vi "Read String.vi"(7 "count (-1: rest)":i64=-1 format="%d elements", 8 "error in (no error)":errorcluster, 9 "offset (0)":u64 format="%d bytes", 10 "buffer in":string, 11 "Pointer in":refnum<class "Pointer.lvclass">) -> (0 "error out":errorcluster, 1 "offset out":u64 format="%d bytes", 2 "buffer out":string, 3 "Pointer out":refnum<class "Pointer.lvclass">)   [LabVIEW 2027, in "Memory Manager.lvlib" / "Pointer.lvclass"]
doc: "Reads <b>count</b> bytes from the address specified by <b>pointer + offset</b> into the provided <b>buffer</b>."
uses:
  Pointer.lvclass
  Read (No Check) String.vi
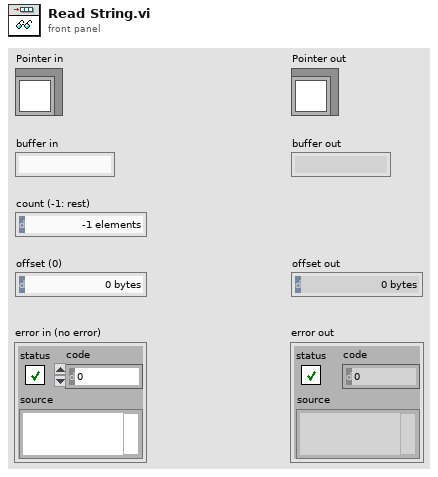
[diagram p1: front panel]
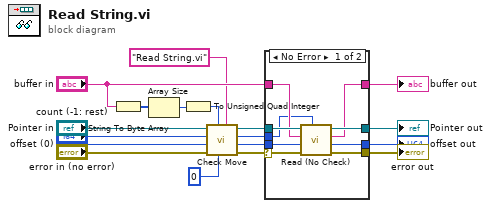
[diagram p0: block diagram]
diagram:
  n1 = String To Byte Array(string="buffer in") -> (unsigned byte array=w14:u8[])
  n2 = Array Size(array=w14) -> (size(s)=w13:i32)
  n3 = To Unsigned Quad Integer(1:w13) -> (0:w7:u64)
  n4 = call "Check Move.vi"("source vi name"="Read String.vi", "count power of 2"=u8 0, "buffer count"=w7, "error in (no error)"="error in (no error)", "offset (0)"="offset (0)", "move count (-1: rest)"="count (-1: rest)", "Pointer in"="Pointer in") -> ("error out"=w10:errorcluster, "offset"=w9:u64, "count"=w8:u64, "Pointer out"=w11:refnum<class "Pointer.lvclass">)  [unwired: 1 in]
  n5 = case shown="No Error" w10 {
    selector: w10 -> [w27 w30]
    tunnel: w11 -> [w25 w29]
    tunnel: w9 -> [w26 w31]
    tunnel: "buffer in" -> [w20 w28]
    tunnel: [w24 w30] -> w18
    tunnel: [w23 w29] -> w16
    tunnel: [w22 w31] -> w15
    tunnel: [w21 w28] -> w17
    tunnel: w8 -> [w19 _]
    frame No Error {
      n6 = call-poly "Read (No Check).vi"("count"=w19, "error in (no error)"=w27, "offset (0)"=w26, "buffer in"=w20, "Pointer in"=w25) -> ("error out"=w24:errorcluster, "offset out"=w22:u64, "buffer out"=w21:string, "Pointer out"=w23:refnum<class "Pointer.lvclass">)  [unwired: 3 in]
    }
    frame Error {
    }
  }
  "error out" <- w18
  "Pointer out" <- w16
  "buffer out" <- w17
  "offset out" <- w15
